vi "Calculations.orig.vi"(0 "Trial in Progress IN":bool, 1 "DIO":bool[](array[boolean]), 3 "cam_vel_ai_vlt":sgl[](array[numeric]), 5 "Sample Rate(s)":dbl=0.002 format="%.3f", 9 "Time Into Trial IN":dbl, 11 "Trial In Progress IN":T1, 12 "Inter-Trial Interval IN":bool) -> (4 "Data Cluster OUT":T2, 6 "Trial Fraction of 1 Reached?":bool, 8 "Timeout Due to Mouse Not Moving?":bool, 10 "Wall Analog Outputs":sgl[](array[numeric]), 13 "Corridor Reset":bool, 14 "Trial Fraction OUT":dbl, 15 "Inter-Trial Interval Complete?":bool)   [LabVIEW 2018]
uses:
  controls/Data To Save.ctl
  controls/Trial Config Settings.ctl
  <vilib>/ptbypt/NI_PtbyPt.lvlib
panel:
  out "Speed_Time_Length":i32
  out "mean_lat_vel":dbl
  out "mean_for_vel":dbl
  out "Vball":dbl format="%.3f"
  out "lat_vel_array":dbl[](array[numeric])
  out "for_vel_array":dbl[](array[numeric])
  out "Cur_Speed_Ind":i32
  out "A_calib_matrix_row1":dbl[](array[numeric])
  out "A_calib_matrix_row0":dbl[](array[numeric])
  out "lat_ball_motion":dbl
  out "for_ball_motion":dbl
  out "zero_V":dbl[](array[numeric])
  out "step_V":dbl
  out "cam_vel_steps":dbl[](array[numeric])
  # "aClck_DI\nframe_clock_DO\nwhisker_video_ctrl_DO\nlick_signal_DI\nwater_valve_trigger\nlaser_ctrl\nleft_texture_ctrl_DO\nright_texture_ctrl_DO\ntrial_ephys_ctrl_DO\ntrial_iti_ctrl_DO\ntrial_on_ctrl_DO\nephys_clock_DO"
  # "*If Speed_Time_Length = 250\nthen averages are calculated every\n0.5 seconds since 1 data save takes\nplace every 0.002 seconds."
  # "="
  # "="
  # "avg"
  # "mean_for_vel"
  # "for_ball_motion (speed_time_length)"
  # "="
  # "="
  # "avg"
  # "mean_lat_vel"
  # "lat_ball_motion (speed_time_length)"
  # "cm/s"
  # "cm/s"
  # "2"
  # "2"
  # "="
  # "+"
  # "cm/s"
  # "for_ball_motion"
  # "lat_ball_motion"
  # "Left Wall"
  # "Vdc"
  # "Right Wall"
  # "Vdc"
  # "A_calib(0,0) x cam_vel_steps(0)"
  # "="
  # "A_calib(0,1) x cam_vel_steps(1)"
  # "sum"
  # "cm/s"
  # "A_calib(0,2) x cam_vel_steps(2)"
  # "A_calib(0,3) x cam_vel_steps(3)"
  # "A_calib(1,0) x cam_vel_steps(0)"
  # "="
  # "A_calib(1,1) x cam_vel_steps(1)"
  # "sum"
  # "cm/s"
  # "A_calib(1,2) x cam_vel_steps(2)"
  # "A_calib(1,3) x cam_vel_steps(3)"
  # "minus"
  # "="
  # "round"
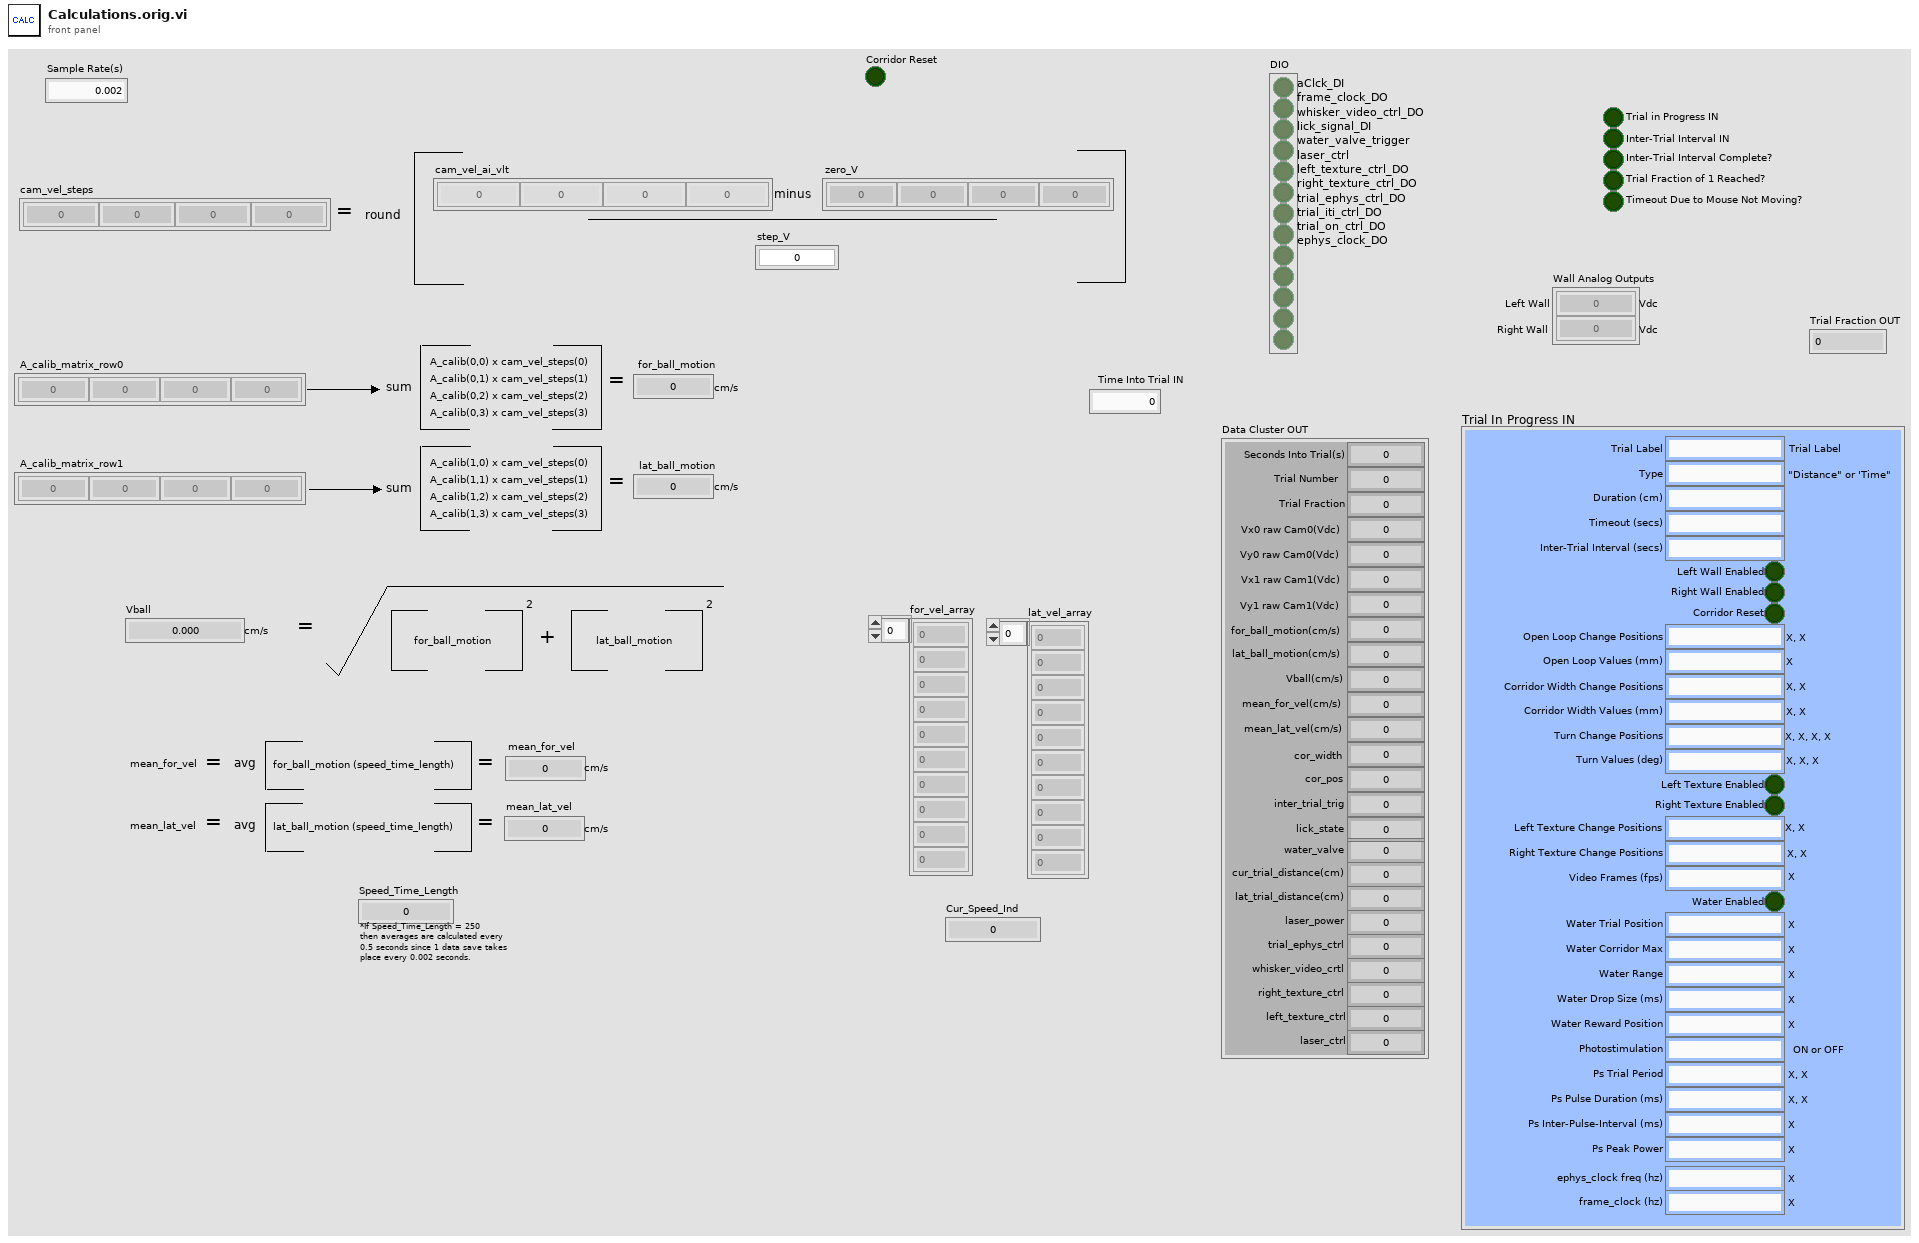
[diagram p1: front panel]
types:
  T1 = typedef "Trial Config Settings.ctl" = cluster{"Trial Label":string, "Type":string, "Timeout (secs)":string, "Inter-Trial Interval (secs)":string, "Left Wall Enabled":bool, "Right Wall Enabled":bool, "Corridor Reset":bool, "Open Loop Change Positions":string, "Open Loop Values (mm)":string, "Corridor Width Change Positions":string, "Corridor Width Values (mm) ":string, "Turn Change Positions":string, "Turn Values (deg)":string, "Left Texture Change Positions":string, "Right Texture Change Positions":string, "Video Frames (fps)":string, "Water Enabled":bool, "Water Trial Position":string, "Photostimulation":string, "Water Corridor Max":string, "Water Range":string, "Water Drop Size (ms)":string, "Water Reward Position":string, "Duration (cm)":string, "Left Texture Enabled":bool, "Right Texture Enabled":bool, "Ps Trial Period":string, "Ps Inter-Pulse-Interval (ms)":string, "Ps Peak Power":string, "Ps Pulse Duration (ms)":string, "ephys_clock freq (hz)":string, "frame_clock (hz)":string}
  T2 = typedef "Data To Save.ctl" = cluster{"Vx0 raw Cam0(Vdc)":sgl, "Vy0 raw Cam0(Vdc)":sgl, "Vx1 raw Cam1(Vdc)":sgl, "Vy1 raw Cam1(Vdc)":sgl, "Seconds Into Trial(s)":dbl, "cor_width":sgl, "cor_pos":sgl, "for_ball_motion(cm/s)":sgl, "lat_ball_motion(cm/s)":sgl, "Vball(cm/s)":sgl, "mean_for_vel(cm/s)":sgl, "mean_lat_vel(cm/s)":sgl, "Trial Fraction":dbl, "Trial Number":i16, "inter_trial_trig":i16, "lick_state":i16, "water_valve":i16, "cur_trial_distance(cm)":dbl, "lat_trial_distance(cm)":dbl, "laser_power":dbl, "trial_ephys_ctrl":i16, "whisker_video_crtl":i16, "right_texture_ctrl":i16, "left_texture_ctrl":i16, "laser_ctrl":i16}
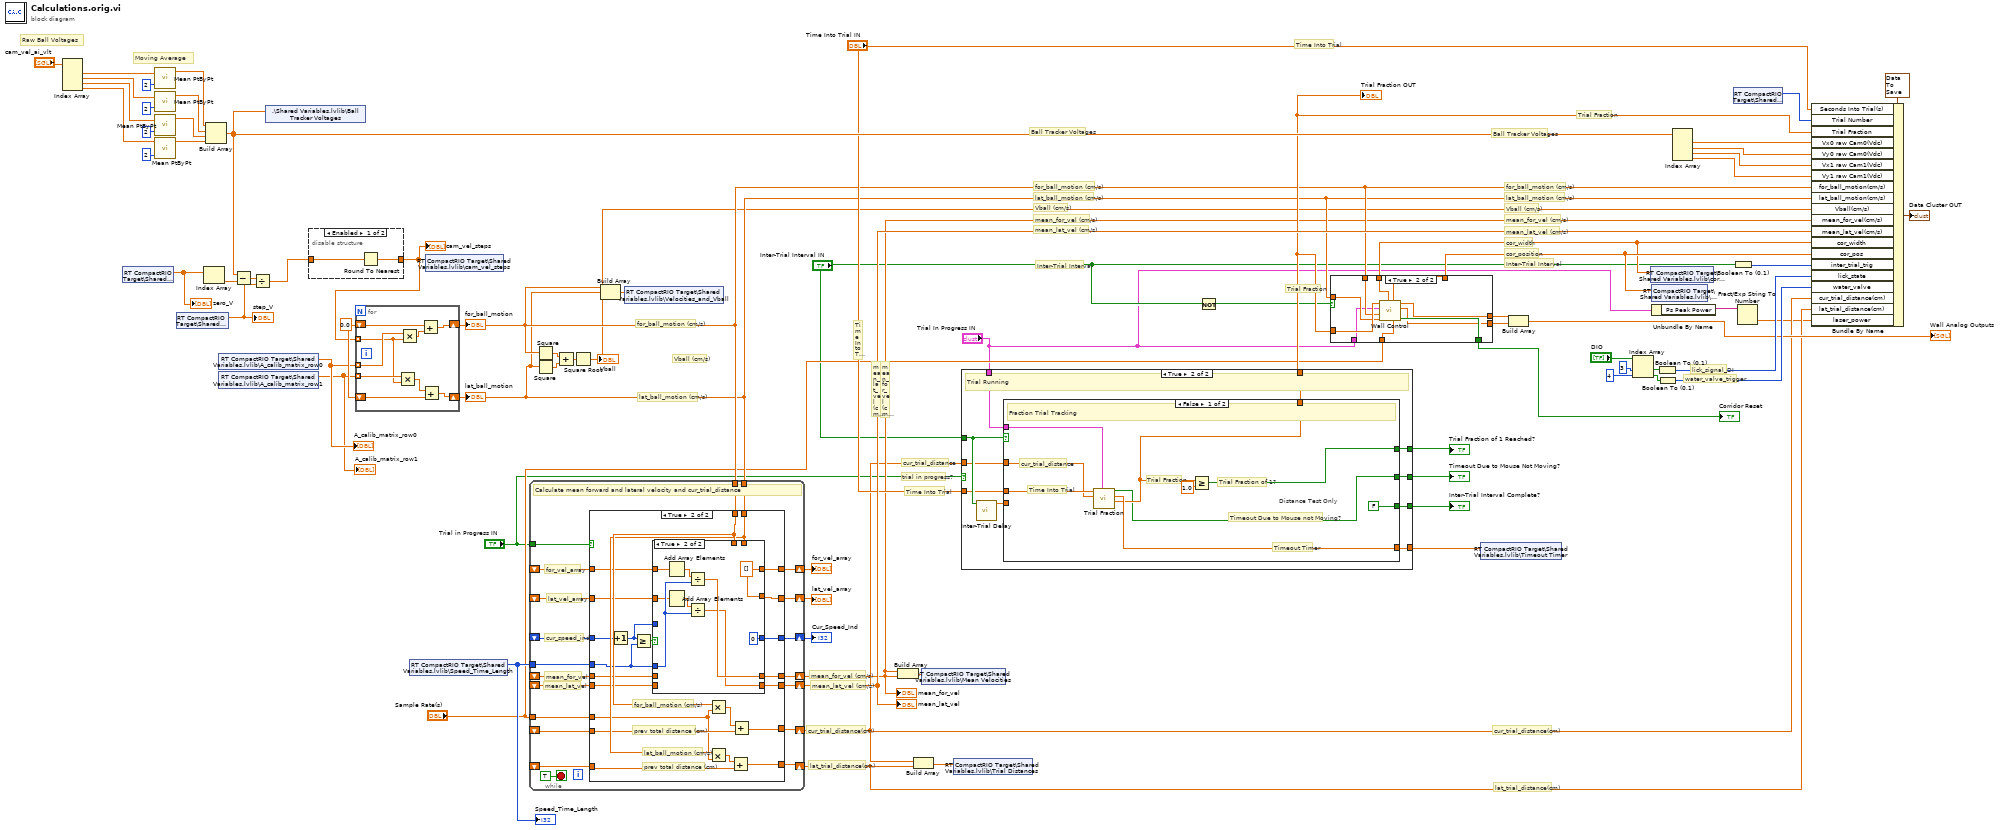
[diagram p0: block diagram]
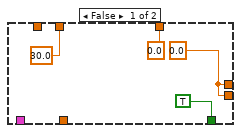
[diagram p2: hidden frame]
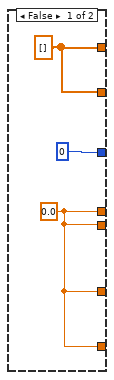
[diagram p3: hidden frame]
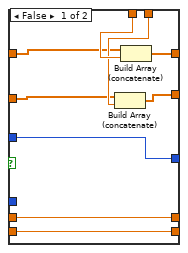
[diagram p4: hidden frame]
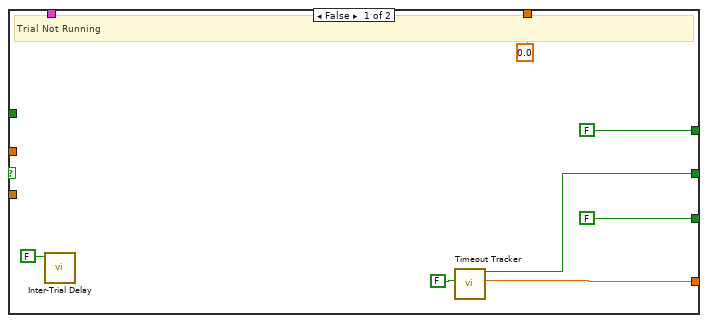
[diagram p5: hidden frame]
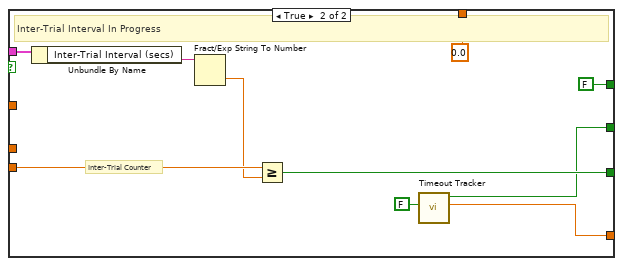
[diagram p6: hidden frame]
diagram:
  w74 = 0.0
  # "Trial Fraction"
  # "lat_trial_distance(cm)"
  # "mean_for_vel (cm/s)"
  # "mean_lat_vel (cm/s)"
  # "cur_trial_distance(cm)"
  # "trial in progress?"
  # "for_ball_motion (cm/s)"
  # "lat_ball_motion (cm/s)"
  # "mean_lat_vel (cm/s)"
  # "mean_for_vel (cm/s)"
  # "Vball (cm/s)"
  # "lat_trial_distance(cm)"
  # "Inter-Trial Interval"
  # "cur_trial_distance(cm)"
  # "mean_for_vel (cm/s)"
  # "mean_lat_vel (cm/s)"
  # "Time Into Trial"
  # "Time Into Trial"
  # "cur_trial_distance"
  # "Vball (cm/s)"
  # "for_ball_motion (cm/s)"
  # "lat_ball_motion (cm/s)"
  # "Inter-Trial Interval"
  # "cor_position"
  # "cor_width"
  # "Ball Tracker Voltages"
  # "Time Into Trial"
  # "Ball Tracker Voltages"
  # "for_ball_motion (cm/s)"
  # "lat_ball_motion (cm/s)"
  # "mean_lat_vel (cm/s)"
  # "mean_for_vel (cm/s)"
  # "Vball (cm/s)"
  # "Trial Fraction"
  # "water_valve_trigger"
  # "lick_signal_DI"
  # "Moving Average"
  # "Raw Ball Voltages"
  n1 = Index Array(array="cam_vel_ai_vlt") -> (element #1=w51:sgl, element #2=w50:sgl, element #3=w49:sgl, element #4=w48:sgl)  [unwired: 4 in]
  n2 = shared-variable "RT CompactRIO Target\\Shared Variables.lvlib\\zero_V"() -> (w70:dbl[])  [unwired: 1 in, 1 out]
  "zero_V" <- w70
  n3 = call <vilib>:"Mean PtByPt.vi"("x"=w51, "sample length"=2) -> ("mean"=w46:dbl)  [unwired: 2 in, 1 out]
  n4 = call <vilib>:"Mean PtByPt.vi"("x"=w50, "sample length"=2) -> ("mean"=w55:dbl)  [unwired: 2 in, 1 out]
  n5 = call <vilib>:"Mean PtByPt.vi"("x"=w49, "sample length"=2) -> ("mean"=w54:dbl)  [unwired: 2 in, 1 out]
  n6 = call <vilib>:"Mean PtByPt.vi"("x"=w48, "sample length"=2) -> ("mean"=w53:dbl)  [unwired: 2 in, 1 out]
  n7 = shared-variable "RT CompactRIO Target\\Shared Variables.lvlib\\step_V"() -> (w69:dbl)  [unwired: 1 in, 1 out]
  "step_V" <- w69
  n8 = Index Array(array=w70) -> (element=w72:dbl)  [unwired: 1 in]
  n9 = Build Array(w46, w55, w54, w53) -> (w47:dbl[])
  n10 = shared-variable "RT CompactRIO Target\\Shared Variables.lvlib\\A_calib_matrix_row0"() -> (w68:dbl[])  [unwired: 1 in, 1 out]
  "A_calib_matrix_row0" <- w68
  n11 = shared-variable "RT CompactRIO Target\\Shared Variables.lvlib\\A_calib_matrix_row1"() -> (w67:dbl[])  [unwired: 1 in, 1 out]
  "A_calib_matrix_row1" <- w67
  n12 = Subtract ("Subtract.vi")(x=w47, y=w72) -> (x-y=w73:dbl[])
  n13 = Divide(x=w73, y=w69) -> (x/y=w71:dbl[])
  n14 = shared-variable ".\\Shared Variables.lvlib\\Ball Tracker Voltages"(w47) -> ()  [unwired: 1 in, 1 out]
  n15 = disable-structure shown="Enabled" {
    disable-tunnel: w71 -> [w76 w77]
    disable-tunnel: [w75 w77] -> w7
    frame Enabled {
      n16 = Round To Nearest(number=w76) -> (nearest integer value=w75:dbl[])
    }
    frame Disabled {
    }
  }
  "cam_vel_steps" <- w7
  n17 = for {
    tunnel: w68 -> [w86] mode=indexing
    tunnel: w67 -> [w85] mode=indexing
    tunnel: w7 -> [w84] mode=indexing
    shift-right: [w81] -> w23
    shift-left: w74 -> [w82]
    shift-right: [w80] -> w22
    shift-left: w74 -> [w78]
    n18 = Multiply(x=w85, y=w84) -> (x*y=w79:dbl)
    n19 = Multiply(x=w86, y=w84) -> (x*y=w83:dbl)
    n20 = Add(x=w82, y=w83) -> (x+y=w81:dbl)
    n21 = Add(x=w79, y=w78) -> (x+y=w80:dbl)
  }
  "for_ball_motion" <- w23
  "lat_ball_motion" <- w22
  n22 = shared-variable "RT CompactRIO Target\\Shared Variables.lvlib\\Speed_Time_Length"() -> (w20:i32)  [unwired: 1 in, 1 out]
  "Speed_Time_Length" <- w20
  n23 = shared-variable "RT CompactRIO Target\\Shared Variables.lvlib\\cam_vel_steps"(w7) -> ()  [unwired: 1 in, 1 out]
  n24 = while {
    tunnel: w23 -> [w106]
    tunnel: w22 -> [w105]
    shift-right: [w104] -> w14
    shift-left: _ -> [w101]
    shift-right: [w103] -> w13
    shift-left: _ -> [w100]
    shift-right: [w98] -> w12
    shift-left: _ -> [w99]
    shift-right: [w96] -> w61
    shift-left: _ -> [w94]
    shift-right: [w97] -> w21
    shift-left: _ -> [w95]
    tunnel: w20 -> [w93]
    tunnel: "Trial in Progress IN" -> [w88]
    shift-right: [w92] -> w19
    shift-left: _ -> [w91]
    shift-right: [w90] -> w17
    shift-left: _ -> [w89]
    tunnel: "Sample Rate(s)" -> [w87]
    stop <- TRUE stop-if-true
    # "mean_for_vel"
    # "mean_lat_vel"
    # "cur_speed_ind"
    # "lat_vel_array"
    # "for_vel_array"
    # "Calculate mean forward and lateral velocity and cur_trial_distance"
    n25 = case shown="True" w88 {
      tunnel: w106 -> [_ w131]
      tunnel: w105 -> [_ w130]
      tunnel: [w109 w129] -> w104
      tunnel: [w109 w128] -> w103
      tunnel: w101 -> [_ w127]
      tunnel: w100 -> [_ w126]
      tunnel: w99 -> [_ w125]
      tunnel: [0 w124] -> w98
      tunnel: [w107 w123] -> w97
      tunnel: [w107 w122] -> w96
      tunnel: w95 -> [_ w121]
      tunnel: w94 -> [_ w120]
      tunnel: w93 -> [_ w119]
      tunnel: [w107 w118] -> w92
      tunnel: w91 -> [_ w117]
      tunnel: [w107 w116] -> w90
      tunnel: w89 -> [_ w115]
      tunnel: w87 -> [_ w110]
      frame False {
        w109 = dbl[] []
        w107 = 0.0 ("mean_for_vel")
      }
      frame True {
        # "prev total distance (cm)"
        # "lat_ball_motion (cm/s)"
        # "prev total distance (cm)"
        # "for_ball_motion (cm/s)"
        n26 = Increment(x=w125) -> (x+1=w113:i32)
        n27 = Greater Or Equal?(x=w113, y=w119) -> (x >= y?=w114:bool)
        n28 = case shown="True" w114 {
          tunnel: [w139 w149] -> w129
          tunnel: [w137 w149] -> w128
          tunnel: w119 -> [_ w146]
          tunnel: w131 -> [w140 _]
          tunnel: w130 -> [w138 _]
          tunnel: w127 -> [w136 w145]
          tunnel: w126 -> [w135 w144]
          tunnel: [w134 0] -> w124
          tunnel: w113 -> [w134 _]
          tunnel: [w133 w142] -> w123
          tunnel: [w132 w141] -> w122
          tunnel: w121 -> [w133 _]
          tunnel: w120 -> [w132 _]
          frame False {
            n29 = Build Array (concatenate)(w135, w138) -> (w137:dbl[])
            n30 = Build Array (concatenate)(w136, w140) -> (w139:dbl[])
          }
          frame True {
            w149 = dbl[] []
            n31 = Add Array Elements(numeric array=w145) -> (sum=w148:dbl)
            n32 = Add Array Elements(numeric array=w144) -> (sum=w147:dbl)
            n33 = Divide(x=w148, y=w146) -> (x/y=w142:dbl)
            n34 = Divide(x=w147, y=w146) -> (x/y=w141:dbl)
          }
        }
        n35 = Multiply(x=w131, y=w110) -> (x*y=w112:dbl)
        n36 = Multiply(x=w130, y=w110) -> (x*y=w111:dbl)
        n37 = Add(x=w111, y=w115) -> (x+y=w116:dbl)
        n38 = Add(x=w112, y=w117) -> (x+y=w118:dbl)
      }
    }
  }
  "mean_for_vel" <- w21
  "mean_lat_vel" <- w61
  "for_vel_array" <- w14
  "lat_vel_array" <- w13
  "Cur_Speed_Ind" <- w12
  n39 = Square(x=w23) -> (x^2=w26:dbl)
  n40 = Square(x=w22) -> (x^2=w25:dbl)
  n41 = Add(x=w26, y=w25) -> (x+y=w24:dbl)
  n42 = Square Root(x=w24) -> (sqrt(x)=w8:dbl)
  "Vball" <- w8
  n43 = Build Array(w23, w22, w8) -> (w65:dbl[])
  n44 = shared-variable "RT CompactRIO Target\\Shared Variables.lvlib\\Velocities_and_Vball"(w65) -> ()  [unwired: 1 in, 1 out]
  n45 = Build Array(w21, w21) -> (w66:dbl[])
  n46 = Build Array(w19, w17) -> (w18:dbl[])
  n47 = shared-variable "RT CompactRIO Target\\Shared Variables.lvlib\\Mean Velocities"(w66) -> ()  [unwired: 1 in, 1 out]
  n48 = shared-variable "RT CompactRIO Target\\Shared Variables.lvlib\\Trial Distances"(w18) -> ()  [unwired: 1 in, 1 out]
  n49 = case shown="True" "Trial in Progress IN" {
    tunnel: "Inter-Trial Interval IN" -> [_ w165]
    tunnel: "Trial In Progress IN" -> [_ w164]
    tunnel: "Time Into Trial IN" -> [_ w163]
    tunnel: w19 -> [_ w162]
    tunnel: [w155 w161] -> w29
    tunnel: [FALSE w160] -> w31
    tunnel: [FALSE w159] -> w11
    tunnel: [0.0 ("Trial Fraction") w158] -> w30
    tunnel: [w150 w157] -> w10
    frame False {
      # "Trial Not Running"
      n50 = call "Inter-Trial Delay.vi"("Start Inter-Trial Delay?"=FALSE) -> ()  [unwired: 10 in, 1 out]
      n51 = call "Timeout Tracker.vi"("Mouse Not Moving?"=FALSE) -> ("Timeout Timer"=w155:dbl, "Timeout"=w150:bool)  [unwired: 9 in]
    }
    frame True {
      # "Trial Running"
      n52 = call "Inter-Trial Delay.vi"("Start Inter-Trial Delay?"=w165) -> ("Inter-Trial Counter (secs)"=w166:dbl)  [unwired: 10 in]
      n53 = case shown="False" w165 {
        tunnel: [w172 w184] -> w161
        tunnel: w166 -> [_ w183]
        tunnel: w164 -> [w174 w182]
        tunnel: w163 -> [w173 _]
        tunnel: w162 -> [w167 _]
        tunnel: [FALSE w179] -> w160
        tunnel: [w169 FALSE] -> w159
        tunnel: [w170 0.0 ("Trial Fraction")] -> w158
        tunnel: [w168 w176] -> w157
        frame False {
          # "cur_trial_distance"
          # "Timeout Timer"
          # "Distance Test Only"
          # "Timeout Due to Mouse not Moving?"
          # "Time Into Trial"
          # "Trial Fraction of 1?"
          # "Trial Fraction"
          # "Fraction Trial Tracking"
          n54 = call "Trial Fraction.vi"("Trial In Progress IN"=w174, "cur_trial_dist"=w167, "Time into Trial"=w173) -> ("Trial Fraction"=w170:dbl, "Timeout Timer"=w172:dbl, "Timeout?"=w168:bool)  [unwired: 6 in]
          n55 = Greater Or Equal?(x=w170, y=1.0) -> (x >= y?=w169:bool)
        }
        frame True {
          # "Inter-Trial Counter"
          # "Inter-Trial Interval In Progress"
          n56 = Unbundle By Name(w182) -> ("Inter-Trial Interval (secs)"=w181:string)
          n57 = Fract/Exp String To Number(string=w181) -> (number=w180:dbl)  [unwired: 3 in, 1 out]
          n58 = Greater Or Equal?(x=w183, y=w180) -> (x >= y?=w179:bool)
          n59 = call "Timeout Tracker.vi"("Mouse Not Moving?"=FALSE) -> ("Timeout Timer"=w184:dbl, "Timeout"=w176:bool)  [unwired: 9 in]
        }
      }
    }
  }
  "Inter-Trial Interval Complete?" <- w31
  "Trial Fraction of 1 Reached?" <- w11
  "Trial Fraction OUT" <- w30
  "Timeout Due to Mouse Not Moving?" <- w10
  n60 = Not(x="Inter-Trial Interval IN") -> (.not. x?=w3:bool)
  n61 = case shown="True" w3 {
    tunnel: [w189 w199] -> w34
    tunnel: w30 -> [_ w198]
    tunnel: [0.0 w197] -> w28
    tunnel: [30.0 w196] -> w27
    tunnel: w23 -> [_ w195]
    tunnel: w22 -> [_ w194]
    tunnel: [TRUE w193] -> w9
    tunnel: "Sample Rate(s)" -> [_ w192]
    tunnel: [w189 w191] -> w2
    tunnel: "Trial In Progress IN" -> [_ w190]
    frame False {
      w189 = 0.0
    }
    frame True {
      n62 = call "Wall Control.vi"("Sample Rate(s)"=w192, "lat_ball_motion IN"=w194, "for_ball_motion IN"=w195, "Trial In Progress IN"=w190, "Trial Fraction IN"=w198) -> ("Corridor Reset"=w193:bool, "Right Wall Analog Output"=w191:sgl, "Left Wall Analog Output"=w199:sgl, "cor_pos OUT"=w197:dbl, "cor_width OUT"=w196:dbl)  [unwired: 2 in]
    }
  }
  "Corridor Reset" <- w9
  n63 = shared-variable "RT CompactRIO Target\\Shared Variables.lvlib\\Timeout Timer"(w29) -> ()  [unwired: 1 in, 1 out]
  n64 = Build Array(w34, w2) -> (→"Wall Analog Outputs":dbl[])
  n65 = Index Array(array="DIO", index #1=3 ("index"), index #2=4 ("index")) -> (element #1=w41:bool, element #2=w36:bool)
  n66 = shared-variable "RT CompactRIO Target\\Shared Variables.lvlib\\cor_width"(w27) -> ()  [unwired: 1 in, 1 out]
  n67 = shared-variable "RT CompactRIO Target\\Shared Variables.lvlib\\cor_pos"(w28) -> ()  [unwired: 1 in, 1 out]
  n68 = Unbundle By Name("Trial In Progress IN") -> ("Ps Peak Power"=w16:string)
  n69 = Boolean To (0,1)(Boolean=w41) -> (0, 1=w40:i16)
  n70 = Boolean To (0,1)(Boolean=w36) -> (0, 1=w35:i16)
  n71 = Index Array(array=w47) -> (element #1=w44:dbl, element #2=w45:dbl, element #3=w63:dbl, element #4=w62:dbl)  [unwired: 4 in]
  n72 = Boolean To (0,1)(Boolean="Inter-Trial Interval IN") -> (0, 1=w38:i16)
  n73 = shared-variable "RT CompactRIO Target\\Shared Variables.lvlib\\Trial#"() -> (w39:i32)  [unwired: 1 in, 1 out]
  n74 = Fract/Exp String To Number(string=w16) -> (number=w15:dbl)  [unwired: 3 in, 1 out]
  n75 = Bundle By Name(cluster=T2 {"Vx0 raw Cam0(Vdc)"=0.0, "Vy0 raw Cam0(Vdc)"=0.0, "Vx1 raw Cam1(Vdc)"=0.0, "Vy1 raw Cam1(Vdc)"=0.0, "Seconds Into Trial(s)"=0.0, "cor_width"=0.0, "cor_pos"=0.0, "for_ball_motion(cm/s)"=0.0, "lat_ball_motion(cm/s)"=0.0, "Vball(cm/s)"=0.0, "mean_for_vel(cm/s)"=0.0, "mean_lat_vel(cm/s)"=0.0, "Trial Fraction"=0.0, "Trial Number"=0, "inter_trial_trig"=0, "lick_state"=0, "water_valve"=0, "cur_trial_distance(cm)"=0.0, "lat_trial_distance(cm)"=0.0, "laser_power"=0.0, "trial_ephys_ctrl"=0, "whisker_video_crtl"=0, "right_texture_ctrl"=0, "left_texture_ctrl"=0, "laser_ctrl"=0} ("Data"), "Seconds Into Trial(s)"="Time Into Trial IN", "Trial Number"=w39, "Trial Fraction"=w30, "Vx0 raw Cam0(Vdc)"=w44, "Vy0 raw Cam0(Vdc)"=w45, "Vx1 raw Cam1(Vdc)"=w63, "Vy1 raw Cam1(Vdc)"=w62, "for_ball_motion(cm/s)"=w23, "lat_ball_motion(cm/s)"=w22, "Vball(cm/s)"=w8, "mean_for_vel(cm/s)"=w21, "mean_lat_vel(cm/s)"=w61, "cor_width"=w27, "cor_pos"=w28, "inter_trial_trig"=w38, "lick_state"=w40, "water_valve"=w35, "cur_trial_distance(cm)"=w19, "lat_trial_distance(cm)"=w17, "laser_power"=w15) -> (→"Data Cluster OUT":T2)
